vi "gaussmeter read channel.vi"(8 "error in (no error)":errorcluster, 10 "channel":T1, 11 "VISA resource name":refnum<visa-resource-name>="GPIB0::12::INSTR") -> (0 "error out":errorcluster, 2 "magnetic field (T)":dbl, 3 "VISA resource name 2":refnum<visa-resource-name>)   [LabVIEW 2013]
uses:
  gaussmeter channels.ctl
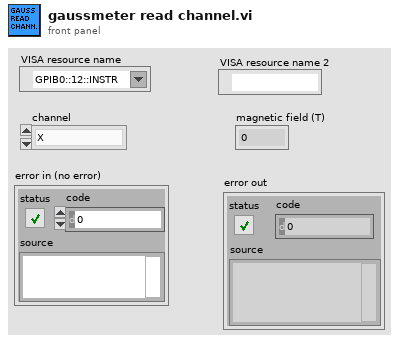
[diagram p1: front panel]
types:
  T1 = typedef "gaussmeter channels.ctl" = enum16{"X", "Y", "Z", "Vec"}
  T2 = typedef "magnet cartesian field.ctl" = cluster{"X (T)":dbl, "Y (T)":dbl, "Z (T)":dbl, "Magnitude (T)":dbl}
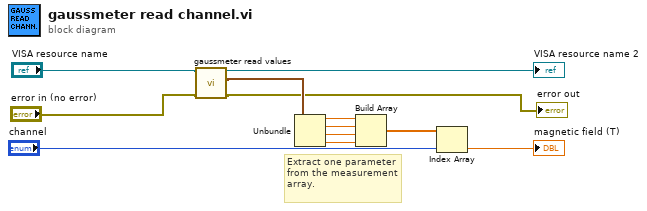
[diagram p0: block diagram]
diagram:
  # "Extract one parameter from the measurement array."
  n1 = call "gaussmeter read values.vi"("error in (no error)"="error in (no error)", "VISA resource name"="VISA resource name") -> ("error out"=→"error out":errorcluster, "gaussmeter reading"=w5:T2, "VISA resource name"=→"VISA resource name 2":refnum<visa-resource-name>)  [unwired: 7 in]
  n2 = Unbundle(w5) -> ("X (T)"=w9:dbl, "Y (T)"=w10:dbl, "Z (T)"=w11:dbl, "Magnitude (T)"=w12:dbl)
  n3 = Build Array(w9, w10, w11, w12) -> (w8:dbl[])
  n4 = Index Array(array=w8, index="channel") -> (element=→"magnetic field (T)":dbl)
